vi "Create Multiple Channels.vi"(7 "Icons":string[](array[string]), 8 "error in":errorcluster, 9 "Channel Descriptions":string[](array[string]), 10 "Channel Names":string[](array[string]), 11 "Item Ref in":T1 format="%.0x") -> (0 "error out":errorcluster)   [LabVIEW 2018, in "NI-XNET Monitor System Explorer.lvlib"]
uses:
  NI-XNET Monitor System Explorer.lvlib
  <vilib>/NI Veristand/Custom Device API/Custom Device Item Ref.ctl
  <vilib>/NI Veristand/Custom Device API/Custom Device Channel.ctl
  <vilib>/NI Veristand/Custom Device API/Custom Device Channel Type.ctl
  <vilib>/NI Veristand/Custom Device API/Custom Device API.lvlib
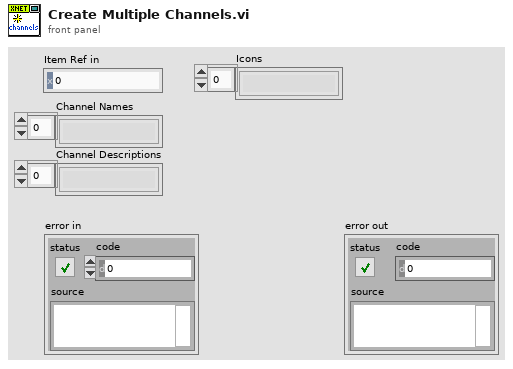
[diagram p1: front panel]
types:
  T1 = typedef "Custom Device API.lvlib/Custom Device Item Ref.ctl" = u64
  T2 = typedef "Custom Device API.lvlib/Custom Device Channel.ctl" = cluster{"Type":T3, "Units":string, "Default Value":dbl, "Faultable":bool, "Scalable":bool}
  T3 = typedef "Custom Device API.lvlib/Custom Device Channel Type.ctl" = enum16{"Input", "Output"}
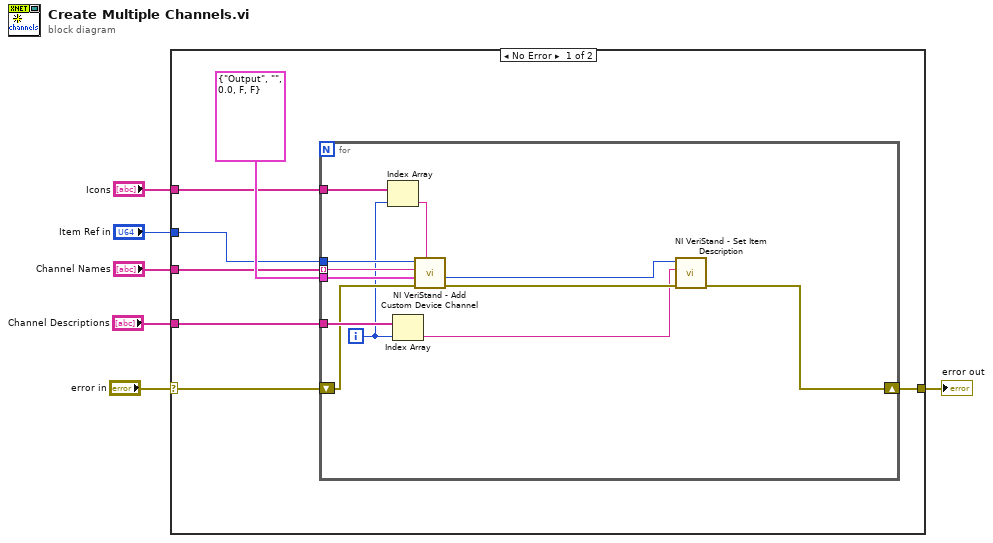
[diagram p0: block diagram]
diagram:
  n1 = case shown="No Error" "error in" {
    selector: "error in" -> [w7 w26]
    tunnel: "Channel Descriptions" -> [w12 _]
    tunnel: "Icons" -> [w11 _]
    tunnel: "Channel Names" -> [w10 _]
    tunnel: [w9 w26] -> w3
    tunnel: "Item Ref in" -> [w8 _]
    frame No Error {
      n2 = for {
        tunnel: w8 -> [w25]
        tunnel: w10 -> [w21] mode=indexing
        tunnel: w11 -> [w16]
        tunnel: w12 -> [w19]
        tunnel: T2 {"Type"=enum."Output", "Units"="", "Default Value"=0.0, "Faultable"=FALSE, "Scalable"=FALSE} ("Channel") -> [w18]
        shift-right: [w22] -> w9
        shift-left: w7 -> [w17]
        i -> [w14]
        n3 = Index Array "Index Array"(array=w16, index=w14) -> (element=w15:string)
        n4 = Index Array "Index Array"(array=w19, index=w14) -> (element=w20:string)
        n5 = call <vilib>:"NI VeriStand - Add Custom Device Channel.vi"("GUID (Default Channel)"=w15, "error in (no error)"=w17, "Channel"=w18, "Channel Name"=w21, "Parent Ref in"=w25) -> ("error out"=w23:errorcluster, "Channel Ref"=w24:T1)  [unwired: 3 in, 2 out]
        n6 = call <vilib>:"NI VeriStand - Set Item Description.vi"("error in (no error)"=w23, "Description"=w20, "Item Ref in"=w24) -> ("error out"=w22:errorcluster)  [unwired: 6 in, 2 out]
      }
    }
    frame Error {
    }
  }
  "error out" <- w3
